vi "Read Executor Number.vi"(8 "error in (no error)":errorcluster, 11 "Job in":refnum<class "Job.lvclass">) -> (0 "error out":errorcluster, 2 "Executor Number":i32, 3 "Job out":refnum<class "Job.lvclass">)   [LabVIEW 2014, in "Job.lvclass"]
uses:
  Job.lvclass
  Job.lvclass/Job.ctl
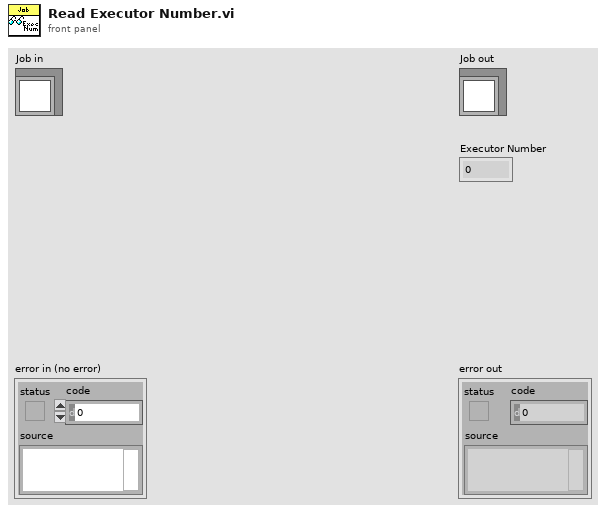
[diagram p1: front panel]
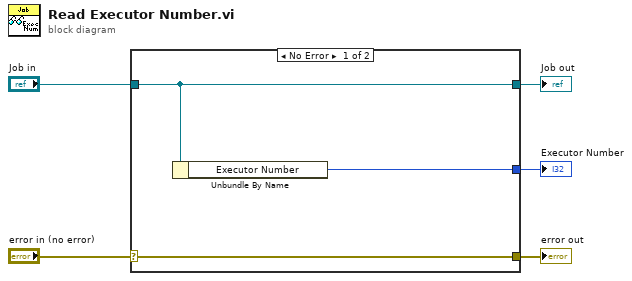
[diagram p0: block diagram]
diagram:
  n1 = case shown="No Error" "error in (no error)" {
    selector: "error in (no error)" -> [w8 w9]
    tunnel: [w8 w9] -> w4
    tunnel: [w7 w10] -> w2
    tunnel: "Job in" -> [w7 w10]
    tunnel: [w6 _] -> w1
    frame No Error {
      n2 = Unbundle By Name(w7) -> ("Executor Number"=w6:i32)
    }
    frame Error {
    }
  }
  "error out" <- w4
  "Job out" <- w2
  "Executor Number" <- w1
